vi "Set BackColor.vi"(8 "error in (no error)":errorcluster caption="错误输入（无错误）", 10 "BackColor":refnum<k24>, 11 "ToolStripLabel 输入":refnum<class "ToolStripLabel.lvclass"> caption="DNL_LabVIEW Object in") -> (0 "error out":errorcluster caption="错误输出", 3 "ToolStripLabel 输出":refnum<class "ToolStripLabel.lvclass"> caption="DNL_LabVIEW Object out")   [LabVIEW 2013, in "ToolStripLabel.lvclass"]
uses:
  ToolStripLabel.lvclass
  System.Drawing
  ToolStripLabel.lvclass/ToolStripLabel.ctl
  System.Windows.Forms
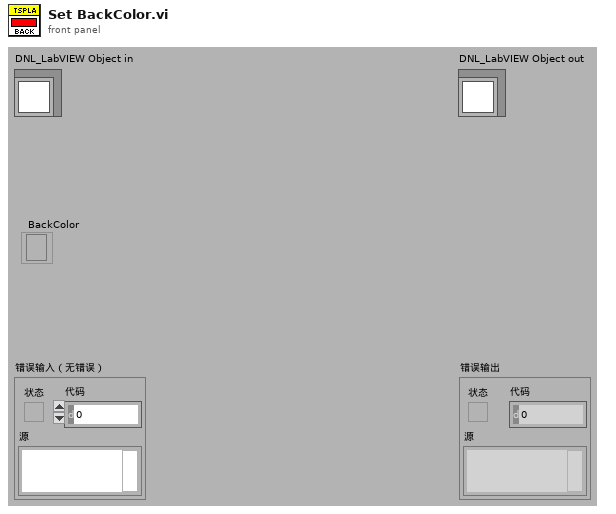
[diagram p1: front panel]
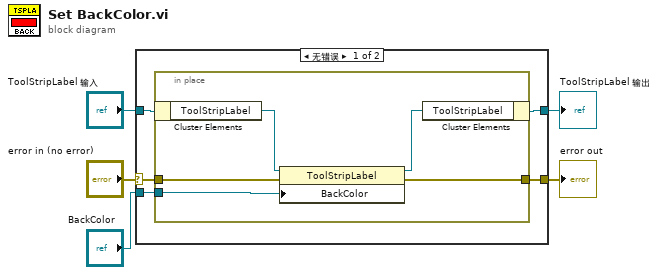
[diagram p0: block diagram]
diagram:
  n1 = case shown="无错误" "error in (no error)" {
    selector: "error in (no error)" -> [w9 w17]
    tunnel: [w8 w17] -> w4
    tunnel: [w7 w16] -> w2
    tunnel: "ToolStripLabel 输入" -> [w10 w16]
    tunnel: "BackColor" -> [w6 _]
    frame No Error {
      n2 = in-place {
        in-place-border: w9 -> [w13]
        in-place-border: [w12] -> w8
        in-place-border: w6 -> [w11]
        n3 = in-place-cluster #1(w10) -> ("ToolStripLabel"=w15:refnum<k24>)
        n4 = property class="ToolStripLabel"(reference=w15, error in=w13, "BackColor"=w11) -> (reference out=w14:refnum<k24>, error out=w12:errorcluster)
        n5 = in-place-cluster #1("ToolStripLabel"=w14) -> (w7:refnum<class "ToolStripLabel.lvclass">)
      }
    }
    frame Error {
    }
  }
  "error out" <- w4
  "ToolStripLabel 输出" <- w2
